vi "Oven_Parameters_Report.vi"(8 "error in (no error)":errorcluster) -> (0 "error out":errorcluster)   [LabVIEW 2017]
uses:
  <vilib>/addons/database/Connection.llb/DB Tools Open Connec (Path).vi
  <vilib>/addons/database/Connection.llb/Conn Execute.vi
  <vilib>/addons/database/Recordset.llb/Rec Fetch Recordset Data (R).vi
  <vilib>/addons/database/Recordset.llb/Rec Destroy - Connection.vi
  <vilib>/Math Plots/3D Math Plots/3D Pie/3D Pie Datatype/Public/Plot Helper (Vector).vi
  <vilib>/addons/database/NI_Database_API.lvlib
  <vilib>/Math Plots/3D Math Plots/3D Pie/3D Pie Datatype/3D Pie Datatype.lvclass
panel:
  out "condition":string
  out "Text.Text 2":string
  in  "Get Rport":bool
  out "Station list":string[](array[string])
  out "Station size":i32
  in  "Tab Control":enum32{"Data"}(tab)
  out "Table":string[][](table)
  in  "To Date":timestamp format="%<%Y-%m-%d>T"
  out "Station Count":i32
  in  "Cancel Button - Archive":bool
  in  "Download 2":bool
  in  "Get Rport 2":bool
  in  "Shift":string(combo)
  in  "Station":string(combo)
  in  "Plan Date":timestamp format="%<%Y-%m-%d>T"
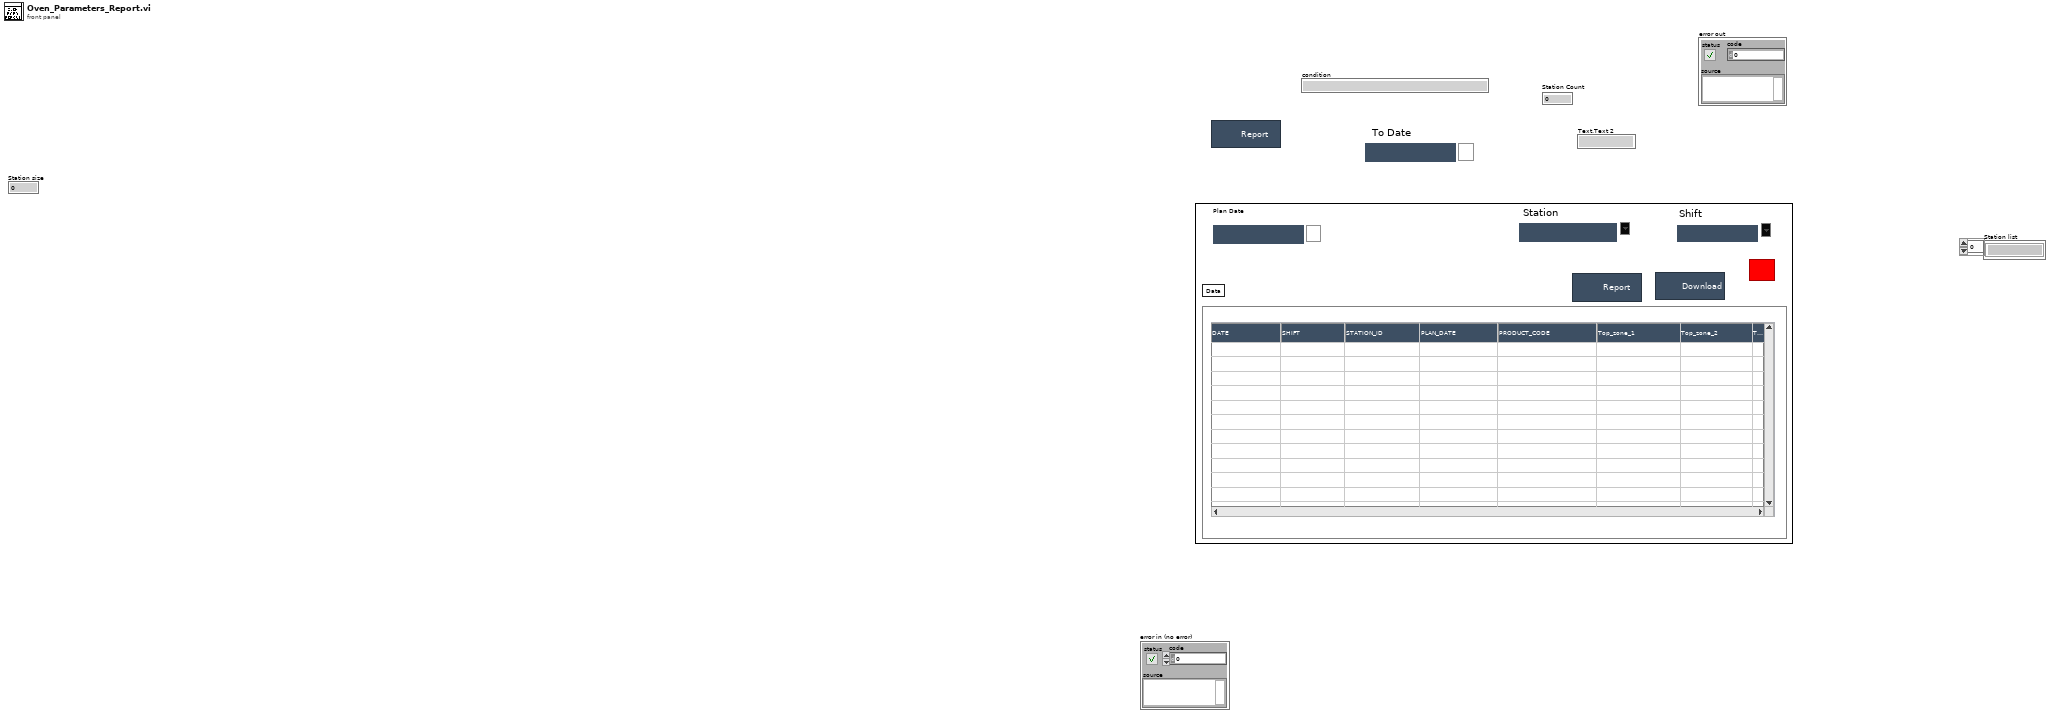
[diagram p1: front panel]
types:
  T1 = typedef "NI_Database_API.lvlib/Conn ObjectReference.ctl" = refnum<k1>
  T2 = typedef "NI_Database_API.lvlib/Rec ObjectReference.ctl" = refnum<k1>
  T3 = enum32{"invalid app kind", "Development System", "Run Time System", "Student Edition", "Embedded LabVIEW", "Evaluation", "Custom"}
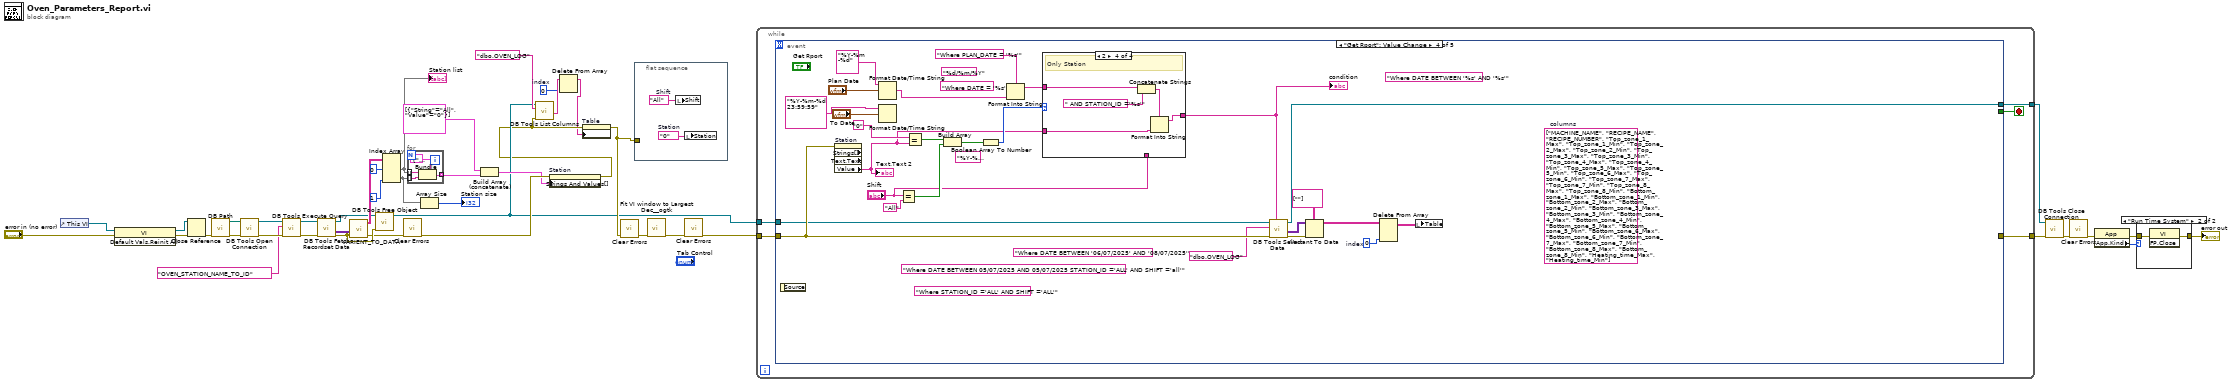
[diagram p0: block diagram]
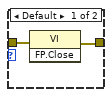
[diagram p2: hidden frame]
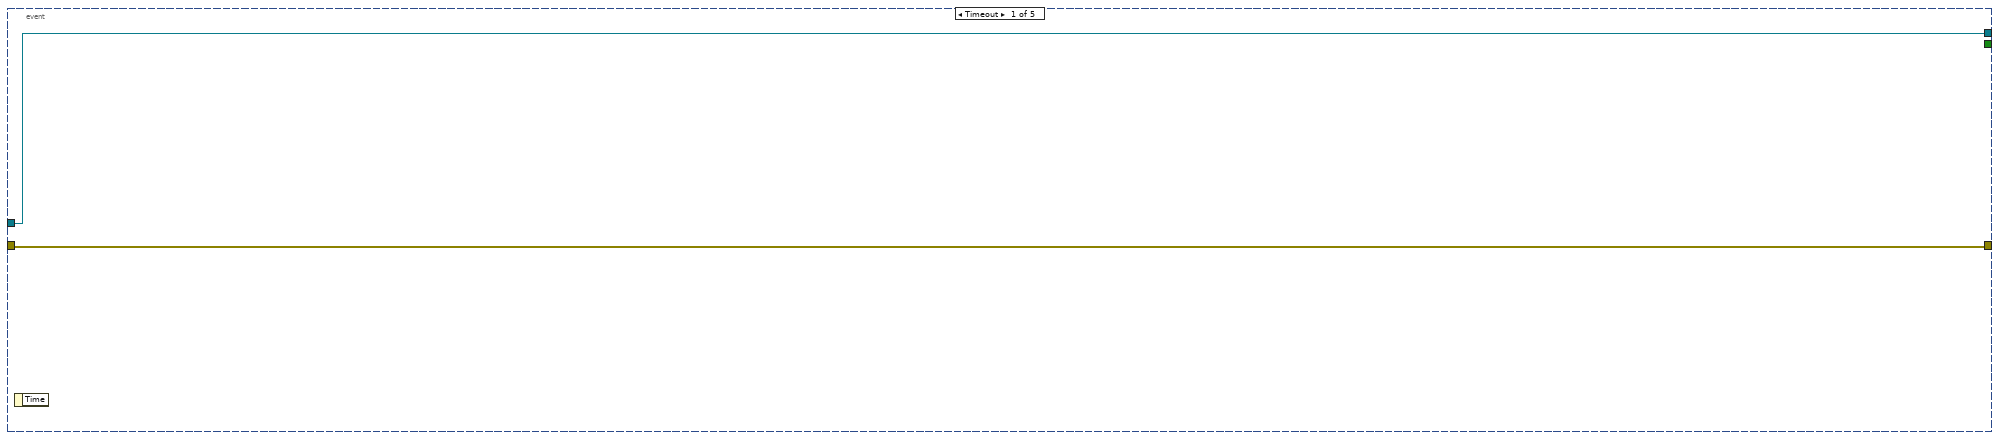
[diagram p3: hidden frame]
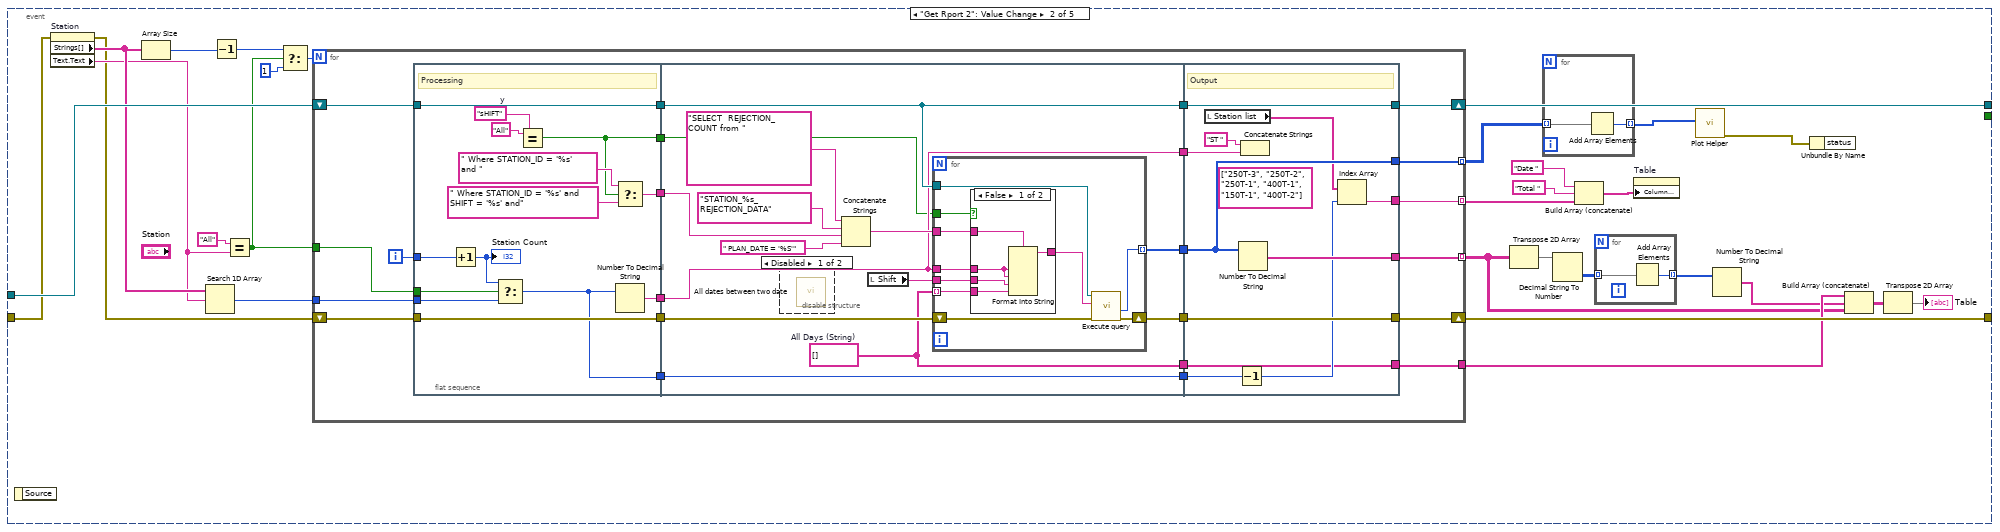
[diagram p4: hidden frame]
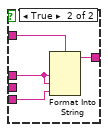
[diagram p6: hidden frame]
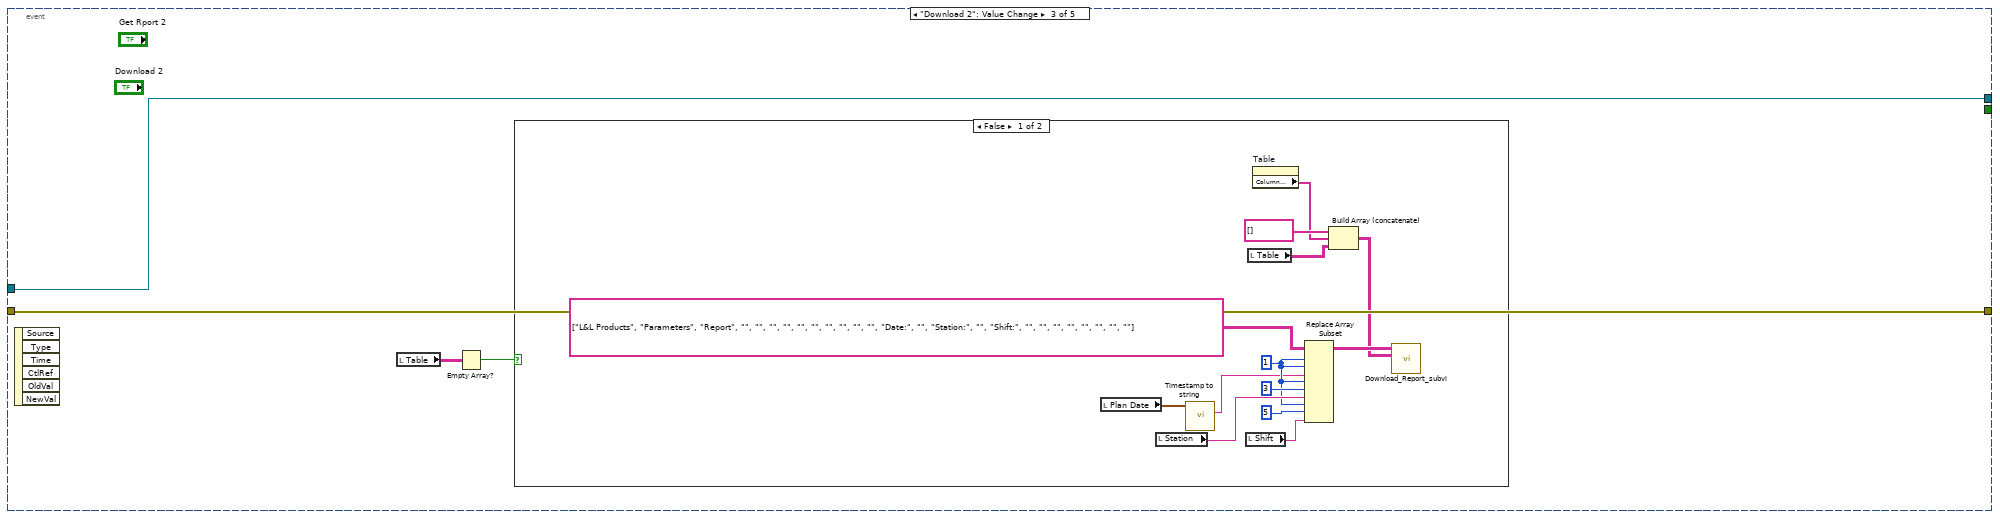
[diagram p7: hidden frame]
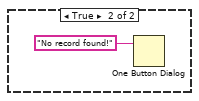
[diagram p8: hidden frame]
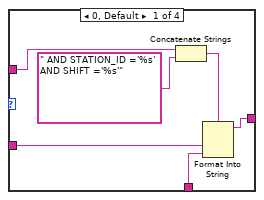
[diagram p9: hidden frame]
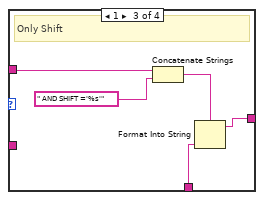
[diagram p11: hidden frame]
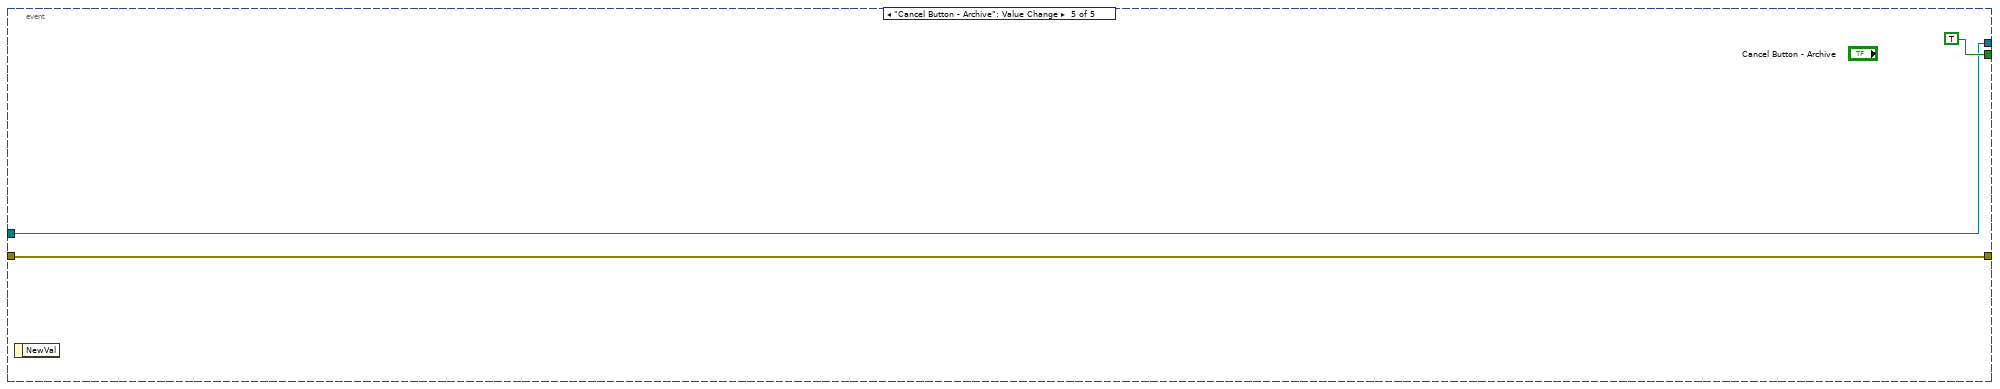
[diagram p12: hidden frame]
diagram:
  w2 = 0  # index
  n1 = control-ref of="This VI"() -> (w36:refnum<vi>)
  n2 = invoke class="VI" method="Default Vals.Reinit All"(reference=w36, error in="error in (no error)") -> (reference out=w34:refnum<vi>, error out=w35:errorcluster)  [unwired: 1 in, 1 out]
  n3 = Close Reference(reference=w34, error in (no error)=w35) -> (error out=w33:errorcluster)
  n4 = call "DB Path.vi"("error in"=w33) -> ("error out"=w32:errorcluster, "DB Path"=w31:path)  [unwired: 9 in]
  n5 = call-poly <vilib>:"DB Tools Open Connection.vi"("error in (no error)"=w32, "connection information"=w31) -> ("error out"=w20:errorcluster, "connection reference"=w21:T1)  [unwired: 6 in]
  n6 = call-poly <vilib>:"DB Tools Execute Query.vi"("error in (no error)"=w20, "SQL query"="OVEN_STATION_NAME_TO_ID", "connection reference"=w21) -> ("error out"=w29:errorcluster, "recordset reference"=w30:T2)  [unwired: 5 in]
  n7 = call-poly <vilib>:"DB Tools Fetch Recordset Data.vi"("error in (no error)"=w29, "recordset reference"=w30) -> ("error out"=w24:errorcluster, "recordset data"=w28:variant[][], "recordset reference out"=w22:T2)  [unwired: 3 in]
  n8 = call "VARIENT_TO_DATA.vi"("data"=w28, "error in (no error)"=w24) -> ("Table"=w25:string[][], "error out"=w23:errorcluster)  [unwired: 7 in]
  n9 = call-poly <vilib>:"DB Tools Free Object.vi"("error in (no error)"=w24, "recordset reference"=w22) -> ("connection reference"=w5:T1)  [unwired: 8 in, 1 out]
  n10 = Index Array(array=w25, index (col) #1=0 ("index (row)"), index (col) #2=1 ("index (col)")) -> (element #1=w12:string[], element #2=w15:string[])  [unwired: 2 in]
  "Station list" <- w12
  n11 = call <vilib>:"Clear Errors.vi"("error in (no error)"=w23) -> ("error out"=w17:errorcluster)  [unwired: 5 in, 1 out]
  n12 = for {
    tunnel: w12 -> [w47] mode=indexing
    tunnel: w15 -> [w46] mode=indexing
    tunnel: [w44] -> w16 mode=indexing
    n13 = Bundle(cluster=cluster{"String":string, "Value":string} {"String"="", "Value"=""}, "String"=w47, "Value"=w46) -> (w44:cluster{"String":string, "Value":string})
  }
  n14 = Array Size(array=w15) -> (size(s)=→"Station size":i32)
  n15 = Build Array (concatenate)(cluster{"String":string, "Value":string}[] [{"String"="All", "Value"="0"}] ("array"), w16) -> (w8:cluster{"String":string, "Value":string}[])
  n16 = property on="Station" class="CmbBox"(error in=w17, "Strings And Values[]"=w8) -> (error out=w4:errorcluster)  [unwired: 1 in, 1 out]
  n17 = call <vilib>:"DB Tools List Columns.vi"("error in (no error)"=w4, "table"="dbo.OVEN_LOG", "connection reference"=w5) -> ("columns"=w3:string[])  [unwired: 1 in, 3 out]
  n18 = Delete From Array(array=w3, index=w2) -> (array with subset deleted=w1:string[])  [unwired: 1 in, 1 out]
  n19 = property on="Table" class="Tbl (strict)"(error in=w4, "Column Headers[]"=w1) -> (error out=w7:errorcluster)  [unwired: 1 in, 1 out]
  n20 = call <vilib>:"Clear Errors.vi"("error in (no error)"=w7) -> ("error out"=w13:errorcluster)  [unwired: 5 in, 1 out]
  n21 = flat-sequence {
    tunnel: w7 -> [_]
    frame #0 {
      w48 = "0"  # Station
      w49 = "All"  # Shift
      n22 = local write "Shift"(w49) -> ()
      n23 = local write "Station"(w48) -> ()
    }
  }
  n24 = call <userlib>:"Fit VI window to Largest Dec__ogtk.vi"("error in (no error)"=w13) -> ("error out"=w10:errorcluster)  [unwired: 5 in, 1 out]
  n25 = call <vilib>:"Clear Errors.vi"("error in (no error)"=w10) -> ("error out"=w9:errorcluster)  [unwired: 5 in, 1 out]
  n26 = while {
    tunnel: w9 -> [w51]
    tunnel: w5 -> [w50]
    tunnel: [w53] -> w39
    tunnel: [w52] -> w38
    stop <- w54 stop-if-true
    n27 = event shown="[3] \"Get Rport\": Value Change" {
      selector: _ -> [_ _ _ _ _]
      dyn-events: _ -> [_ _ _ _ _]
      timeout: _ -> [_ _ _ _ _]
      tunnel: w50 -> [w55 w85 w174 w209 w233]
      tunnel: [_ _ _ _ TRUE] -> w54
      tunnel: [w56 w83 w173 _ w232] -> w53
      tunnel: [w55 w84 w174 w207 w233] -> w52
      tunnel: w51 -> [w56 w58 w173 w210 w232]
      event Timeout {
        n28 = event-data() -> ()  [unwired: 1 in, 1 out]
      }
      event "Get Rport 2": Value Change {
        n29 = event-data() -> ()  [unwired: 1 in, 1 out]
        n30 = property on="Station" class="CmbBox"(error in=w58) -> (error out=w57:errorcluster, "Strings[]"=w64:string[], "Text.Text"=w59:string)  [unwired: 1 in, 1 out]
        n31 = Array Size(array=w64) -> (size(s)=w79:i32)
        n32 = Search 1D Array(1D array=w64, element=w59) -> (index of element=w76:i32)  [unwired: 1 in]
        n33 = Decrement(x=w79) -> (x-1=w78:i32)
        n34 = Equal?(x="All", y=w59) -> (x = y?=w77:bool)
        n35 = Select(t=w78, s=w77, f=1) -> (s? t:f=w81:i32)
        n36 = for {
          N: w81 -> [_]
          shift-right: [w105] -> w84
          shift-left: w85 -> [w112]
          shift-right: [w106] -> w83
          shift-left: w57 -> [w111]
          tunnel: w77 -> [w110]
          tunnel: w76 -> [w109]
          tunnel: [w107] -> w60 mode=indexing
          tunnel: [w97] -> w69 mode=indexing
          tunnel: [w96] -> w72
          tunnel: [w90] -> w61 mode=indexing
          i -> [w108]
          n37 = flat-sequence {
            tunnel: [w123] -> w104
            tunnel: [w124] -> w102
            tunnel: [w126] -> w100
            tunnel: [w125] -> w99
            tunnel: w108 -> [w119]
            tunnel: w109 -> [w120]
            tunnel: w110 -> [w121]
            tunnel: w111 -> [w123]
            tunnel: w112 -> [w124]
            tunnel: [w115] -> w93
            tunnel: [w114] -> w91
            tunnel: w104 -> [w133]
            tunnel: [w132] -> w103
            tunnel: w102 -> [w134]
            tunnel: [w134] -> w101
            tunnel: w100 -> [w138]
            tunnel: w99 -> [w130]
            tunnel: [w131] -> w98
            tunnel: [w130] -> w95
            tunnel: [w127] -> w94
            tunnel: w93 -> [w129]
            tunnel: [w128] -> w92
            tunnel: w91 -> [w128]
            tunnel: [w164] -> w107
            tunnel: w103 -> [w166]
            tunnel: [w166] -> w106
            tunnel: [w170] -> w105
            tunnel: w101 -> [w170]
            tunnel: w98 -> [w162]
            tunnel: [w169] -> w97
            tunnel: [w161] -> w96
            tunnel: w95 -> [w168]
            tunnel: w94 -> [w161]
            tunnel: w92 -> [w165]
            tunnel: [w162] -> w90
            frame #0 {
              w113 = "sHIFT"  # y
              # "Processing"
              n38 = Increment(x=w119) -> (x+1=w118:i32)
              "Station Count" <- w118
              n39 = Select(t=w118, s=w121, f=w120) -> (s? t:f=w114:i32)
              n40 = Equal?(x="All", y=w113) -> (x = y?=w115:bool)
              n41 = Select(t=" Where STATION_ID = '%s' and " ("format string"), s=w115, f=" Where STATION_ID = '%s' and SHIFT = '%s' and" ("format string")) -> (s? t:f=w126:string)
              n42 = Number To Decimal String(number=w114) -> (decimal integer string=w125:string)  [unwired: 1 in]
            }
            frame #1 {
              w127 = string[] []  # All Days (String)
              n43 = disable-structure shown="Disabled" {
                frame Disabled {
                  n44 = call "All dates between two date.vi"() -> ()  [unwired: 10 in, 2 out]
                }
                frame Enabled {
                }
              }
              n45 = Concatenate Strings("SELECT  REJECTION_COUNT from " ("format string"), "STATION_%s_REJECTION_DATA", w138, " PLAN_DATE = '%S'" ("string")) -> (w136:string)
              n46 = local read "Shift"() -> (w135:string)
              n47 = for {
                tunnel: w129 -> [w150]
                tunnel: w136 -> [w149]
                tunnel: w130 -> [w148]
                tunnel: w135 -> [w147]
                tunnel: w127 -> [w146] mode=indexing
                tunnel: w134 -> [w144]
                shift-right: [w142] -> w132
                shift-left: w133 -> [w143]
                tunnel: [w141] -> w131 mode=indexing
                n48 = case shown="False" w150 {
                  tunnel: w149 -> [w155 w159]
                  tunnel: w148 -> [w154 w158]
                  tunnel: w147 -> [w153 _]
                  tunnel: w146 -> [w152 w157]
                  tunnel: [w151 w156] -> w145
                  frame False {
                    n49 = Format Into String(format string=w155, w154, w154, w153, w152) -> (resulting string=w151:string)  [unwired: 2 in, 1 out]
                  }
                  frame True {
                    n50 = Format Into String(format string=w159, w158, w158, w157) -> (resulting string=w156:string)  [unwired: 2 in, 1 out]
                  }
                }
                n51 = call "Execute query.vi"("error in (no error)"=w143, "String"=w145, "connection reference"=w144) -> ("error out"=w142:errorcluster, "Production Count"=w141:i32)  [unwired: 3 in, 4 out]
              }
            }
            frame #2 {
              (unwired) string[] ["250T-3", "250T-2", "250T-1", "400T-1", "150T-1", "400T-2"]
              # "Output"
              n52 = local read "Station list"() -> (w160:string[])
              n53 = Decrement(x=w165) -> (x-1=w163:i32)
              n54 = Number To Decimal String(number=w162) -> (decimal integer string=w169:string[])  [unwired: 1 in]
              n55 = Concatenate Strings("ST " ("string"), w168) -> ()  [unwired: 1 out]
              n56 = Index Array(array=w160, index=w163) -> (element=w164:string)
            }
          }
        }
        n57 = Transpose 2D Array(2D array=w69) -> (transposed array=w68:string[][])
        n58 = for {
          tunnel: w61 -> [w87] mode=indexing
          tunnel: [w86] -> w62 mode=indexing
          n59 = Add Array Elements(numeric array=w87) -> (sum=w86:i32)
        }
        n60 = Decimal String To Number(string=w68) -> (number=w67:i32[][])  [unwired: 2 in, 1 out]
        n61 = Build Array (concatenate)("Date ", "Total ", w60) -> (w75:string[])
        n62 = for {
          tunnel: w67 -> [w89] mode=indexing
          tunnel: [w88] -> w66 mode=indexing
          n63 = Add Array Elements(numeric array=w89) -> (sum=w88:i32)
        }
        n64 = property on="Table" class="Tbl (strict)"("Column Headers[]"=w75) -> ()  [unwired: 2 in, 2 out]
        n65 = call-poly <vilib>:"Plot Helper.vi"("x vector"=w62) -> ("error out"=w63:errorcluster)  [unwired: 2 in, 8 out]
        n66 = Number To Decimal String(number=w66) -> (decimal integer string=w65:string[])  [unwired: 1 in]
        n67 = Unbundle By Name(w63) -> ()  [unwired: 1 out]
        n68 = Build Array (concatenate)(w72, w65, w69) -> (w74:string[][])
        n69 = Transpose 2D Array(2D array=w74) -> (transposed array=→"Table":string[][])
      }
      event "Download 2": Value Change {
        n70 = event-data() -> ()  [unwired: 1 in, 6 out]
        n71 = local read "Table"() -> (w172:string[][])
        n72 = Empty Array?(array=w172) -> (empty?=w171:bool)
        n73 = case shown="False" w171 {
          frame False {
            w183 = 1 ("index (row)")
            n74 = local read "Plan Date"() -> (w180:timestamp)
            n75 = local read "Station"() -> (w184:string)
            n76 = call "Timestamp to string.vi"("time stamp"=w180) -> ("Date"=w179:string)  [unwired: 8 in, 2 out]
            n77 = local read "Shift"() -> (w181:string)
            n78 = local read "Table"() -> (w178:string[][])
            n79 = property on="Table" class="Tbl (strict)"() -> ("Column Headers[]"=w175:string[])  [unwired: 2 in, 2 out]
            n80 = Replace Array Subset(array=string[][] [["L&L Products", "Parameters", "Report", "", "", "", "", "", "", "", "", "", ""], ["Date:", "", "Station:", "", "Shift:", "", "", "", "", "", "", "", ""]] ("Column Header Strings[]"), new element #1=w179, index (row) #1=w183, index (col) #1=w183, new element #2=w184, index (row) #2=w183, index (col) #2=3 ("disabled index (col)"), new element #3=w181, index (row) #3=w183, index (col) #3=5 ("disabled index (col)")) -> (w186:string[][])
            n81 = Build Array (concatenate)(string[] [] ("element"), w175, w178) -> (w177:string[][])
            n82 = call "Download_Report_subvi.vi"("Value"=w177, "Column Header Strings[]"=w186) -> ()  [unwired: 9 in, 1 out]
          }
          frame True {
            n83 = One Button Dialog(message="No record found!") -> ()  [unwired: 1 in, 1 out]
          }
        }
      }
      event "Get Rport": Value Change {
        (unwired) "Where DATE BETWEEN '%s' AND '%s'" ("condition")
        (unwired) "Where DATE = '%s'" ("condition")
        (unwired) "%Y-%m-%d %H:%M:%S" ("condition")
        w191 = 0  # index
        (unwired) "%d/%m/%Y" ("time format string (%c)")
        (unwired) "Where DATE BETWEEN 05/07/2025 AND 05/07/2025 STATION_ID ='ALL' AND SHIFT ='all'" ("condition")
        (unwired) "Where STATION_ID ='ALL' AND SHIFT ='ALL'" ("condition")
        (unwired) "Where DATE BETWEEN '06/07/2025' AND '08/07/2025'" ("condition")
        (unwired) string[] ["MACHINE_NAME", "RECIPE_NAME", "RECIPE_NUMBER", "Top_zone_1_Max", "Top_zone_1_Min", "Top_zone_2_Max", "Top_zone_2_Min", "Top_zone_3_Max", "Top_zone_3_Min", "Top_zone_4_Max", "Top_zone_4_Min", "Top_zone_5_Max", "Top_zone_5_Min", "Top_zone_6_Max", "Top_zone_6_Min", "Top_zone_7_Max", "Top_zone_7_Min", "Top_zone_8_Max", "Top_zone_8_Min", "Bottom_zone_1_Max", "Bottom_zone_1_Min", "Bottom_zone_2_Max", "Bottom_zone_2_Min", "Bottom_zone_3_Max", "Bottom_zone_3_Min", "Bottom_zone_4_Max", "Bottom_zone_4_Min", "Bottom_zone_5_Max", "Bottom_zone_5_Min", "Bottom_zone_6_Max", "Bottom_zone_6_Min", "Bottom_zone_7_Max", "Bottom_zone_7_Min", "Bottom_zone_8_Max", "Bottom_zone_8_Min", "Heating_time_Max", "Heating_time_Min"]  # columns
        n84 = event-data() -> ()  [unwired: 1 in, 1 out]
        n85 = property on="Station" class="CmbBox" props=["Strings[]", "Text", "Text", "Value"](error in=w210) -> ("Value"=w199:string)  [unwired: 1 in, 4 out]
        "Text.Text 2" <- w199
        n86 = Format Date/Time String(time format string (%c)="%Y-%m-%d" ("condition"), seconds (now)="Plan Date") -> (date/time string=w196:string)  [unwired: 1 in]
        n87 = Format Date/Time String(time format string (%c)="%Y-%m-%d 23:59:59" ("condition"), seconds (now)="To Date") -> ()  [unwired: 1 in, 1 out]
        n88 = Equal?(x="Shift", y="All" ("x")) -> (x = y?=w203:bool)
        n89 = Equal?(x="0", y=w199) -> (x = y?=w204:bool)
        n90 = Build Array(w204, w203) -> (w202:bool[])
        n91 = Boolean Array To Number(Boolean array=w202) -> (number=w201:u32)
        n92 = Format Into String(format string="Where PLAN_DATE = '%s'" ("condition"), w196) -> (resulting string=w195:string)  [unwired: 2 in, 1 out]
        n93 = case shown="2" w201 {
          tunnel: [w220 w221 w225 w231] -> w194
          tunnel: "Shift" -> [w219 _ w226 _]
          tunnel: w199 -> [w218 _ _ w230]
          tunnel: w195 -> [w217 w221 w224 w229]
          frame 0, Default {
            n94 = Concatenate Strings(w217, " AND STATION_ID ='%s' AND SHIFT ='%s'" ("condition")) -> (w215:string)
            n95 = Format Into String(format string=w215, w218, w219) -> (resulting string=w220:string)  [unwired: 2 in, 1 out]
          }
          frame 3 {
            # "All station and Shift"
          }
          frame 1 {
            # "Only Shift"
            n96 = Concatenate Strings(w224, " AND SHIFT ='%s'" ("condition")) -> (w222:string)
            n97 = Format Into String(format string=w222, w226) -> (resulting string=w225:string)  [unwired: 2 in, 1 out]
          }
          frame 2 {
            # "Only Station"
            n98 = Concatenate Strings(w229, " AND STATION_ID ='%s'" ("condition")) -> (w227:string)
            n99 = Format Into String(format string=w227, w230) -> (resulting string=w231:string)  [unwired: 2 in, 1 out]
          }
        }
        "condition" <- w194
        n100 = call <vilib>:"DB Tools Select Data.vi"("condition"=w194, "error in (no error)"=w210, "table"="dbo.OVEN_LOG", "connection reference"=w209) -> ("error out"=w211:errorcluster, "data"=w212:variant[][], "connection reference out"=w207:T1)  [unwired: 2 in]
        n101 = Variant To Data(error in=w211, type=string[][] [[""]], Variant=w212) -> (data=w193:string[][])  [unwired: 1 out]
        n102 = Delete From Array(array=w193, index (col)=w191) -> (array with subset deleted=w192:string[][])  [unwired: 2 in, 1 out]
        n103 = local write "Table"(w192) -> ()
      }
      event "Cancel Button - Archive": Value Change {
        n104 = event-data() -> ()  [unwired: 1 in, 1 out]
      }
    }
  }
  n105 = call <vilib>:"DB Tools Close Connection.vi"("error in (no error)"=w39, "connection reference"=w38) -> ("error out"=w41:errorcluster)  [unwired: 5 in]
  n106 = call <vilib>:"Clear Errors.vi"("error in (no error)"=w41) -> ("error out"=w40:errorcluster)  [unwired: 5 in, 1 out]
  n107 = property class="App"(error in=w40) -> (error out=w42:errorcluster, "App.Kind"=w43:T3)  [unwired: 1 in, 1 out]
  n108 = case shown="\"Run Time System\"" w43 {
    tunnel: w42 -> [w235 w238]
    tunnel: [w236 w237] -> w37
    frame Default {
      n109 = invoke class="VI" method="FP.Close"(error in=w235) -> (error out=w236:errorcluster)  [unwired: 2 in, 2 out]
    }
    frame "Run Time System" {
      n110 = invoke class="VI" method="FP.Close"(error in=w238) -> (error out=w237:errorcluster)  [unwired: 2 in, 2 out]
    }
  }
  "error out" <- w37
